vi "DetectorClose.vi"(8 "error in (no error)":errorcluster, 11 "Microscope in":refnum<class "Microscope.lvclass">) -> (0 "error out":errorcluster, 3 "Microscope out":refnum<class "Microscope.lvclass">)   [LabVIEW 2012, in "Microscope.lvclass"]
uses:
  classes/Microscope.lvclass
  classes/Microscope.lvclass/Microscope.ctl
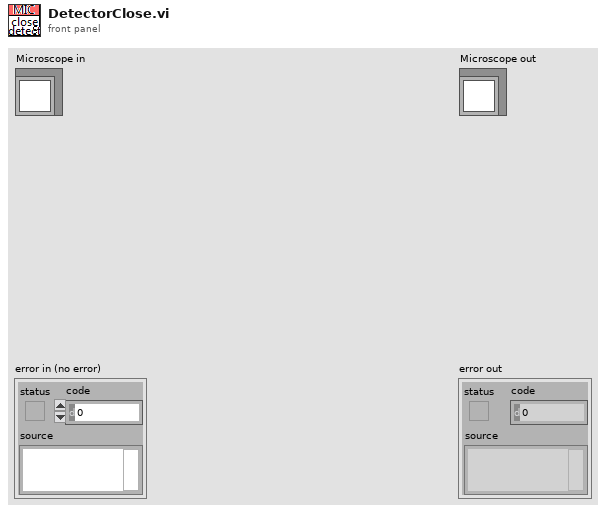
[diagram p1: front panel]
types:
  T1 = typedef "DetectorType.ctl" = enum16{"PMT", "SpectraWiz"}
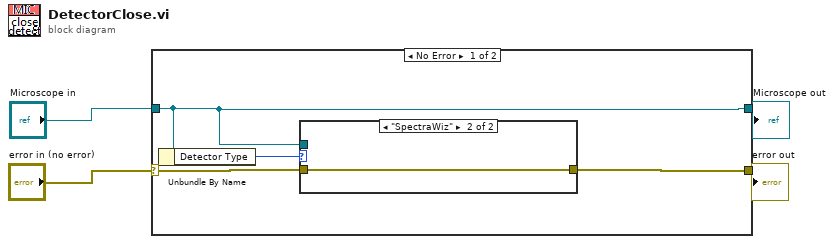
[diagram p0: block diagram]
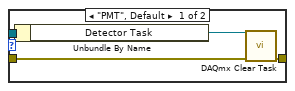
[diagram p2: hidden frame]
diagram:
  n1 = case shown="No Error" "error in (no error)" {
    selector: "error in (no error)" -> [w7 w15]
    tunnel: [w8 w15] -> w3
    tunnel: [w6 w14] -> w1
    tunnel: "Microscope in" -> [w6 w14]
    frame No Error {
      n2 = Unbundle By Name(w6) -> ("Detector Type"=w5:T1)
      n3 = case shown="\"SpectraWiz\"" w5 {
        tunnel: [w11 w13] -> w8
        tunnel: w7 -> [w10 w13]
        tunnel: w6 -> [w9 _]
        frame "PMT", Default {
          n4 = Unbundle By Name(w9) -> ("Detector Task"=w12:refnum<k21>)
          n5 = call <vilib>:"DAQmx Clear Task.vi"("task in"=w12, "error in"=w10) -> ("error out"=w11:errorcluster)  [unwired: 13 in]
        }
        frame "SpectraWiz" {
        }
      }
    }
    frame Error {
    }
  }
  "error out" <- w3
  "Microscope out" <- w1
